vi "Fetch Measurement-Sweep.vi"(8 "error in (no error)":errorcluster, 10 "Measure Call Context in":refnum<class "Measure Call Context.lvclass">, 11 "Sweep fetch measurement control":T1={"Source Ganged Session Out"={"Ganged Config"=enum."Series", "Session List"=[], "Session Mode"=[], "Channel"=[]}, "Load Ganged Session Out"={"Ganged Config"=enum."Series", "Session List"=[], "Session Mode"=[], "Channel"=[]}, "Source sweep values"=[], "Source sweep points"=0, "Load sweep values"=[], "Load sweep points"=0, "Measurement Results"={"Status"="", "Source sweep points"=0, "Load sweep points"=0, "Source sweep values"=[], "Load sweep values"=[], "Source voltages"=[], "Source currents"=[], "Load voltages"=[], "Load currents"=[], "Eload status"=""}, "Load ganged/single"=FALSE, "Source ganged/single"=FALSE, "Source channel name"="", "Load channel name"="", "Source session out"="", "Load session out"="", "Load Source ON/OFF"=enum."SOURCE AND LOAD OFF", "Measurement timeout"=10.0} {"Measurement timeout" format="%.3p"}) -> (0 "error out":errorcluster, 3 "Sweep fetch measurement":T1={"Source Ganged Session Out"={"Ganged Config"=enum."Series", "Session List"=[], "Session Mode"=[], "Channel"=[]}, "Load Ganged Session Out"={"Ganged Config"=enum."Series", "Session List"=[], "Session Mode"=[], "Channel"=[]}, "Source sweep values"=[], "Source sweep points"=0, "Load sweep values"=[], "Load sweep points"=0, "Measurement Results"={"Status"="", "Source sweep points"=0, "Load sweep points"=0, "Source sweep values"=[], "Load sweep values"=[], "Source voltages"=[], "Source currents"=[], "Load voltages"=[], "Load currents"=[], "Eload status"=""}, "Load ganged/single"=FALSE, "Source ganged/single"=FALSE, "Source channel name"="", "Load channel name"="", "Source session out"="", "Load session out"="", "Load Source ON/OFF"=enum."SOURCE AND LOAD OFF", "Measurement timeout"=10.0} {"Measurement timeout" format="%.3p"})   [LabVIEW 2021, in "Sweep_Channel Ganging.lvlib"]
doc: "This vi fetches the measurement for the different configuration of single and ganging also when only source or load is enabled"
uses:
  Controls/Sweep fetch measurement control.ctl
  shared subVIs/ctl/NIDCPower_channel_ganging - ctl - ganged session.ctl
  shared subVIs/ctl/NIDCPower_channel_ganging - ctl - ganged config.ctl
  shared subVIs/ctl/NIDCPower_channel_ganging - ctl - channel mode.ctl
  Measurement Results.ctl
  <vilib>/Plug-In SDKs/Measurements/Measure Call Context/Measure Call Context.lvclass
  <vilib>/Plug-In SDKs/Measurements/Measure Call Context/Accessor/Is Canceled.vi
  Sweep_Channel Ganging.lvlib
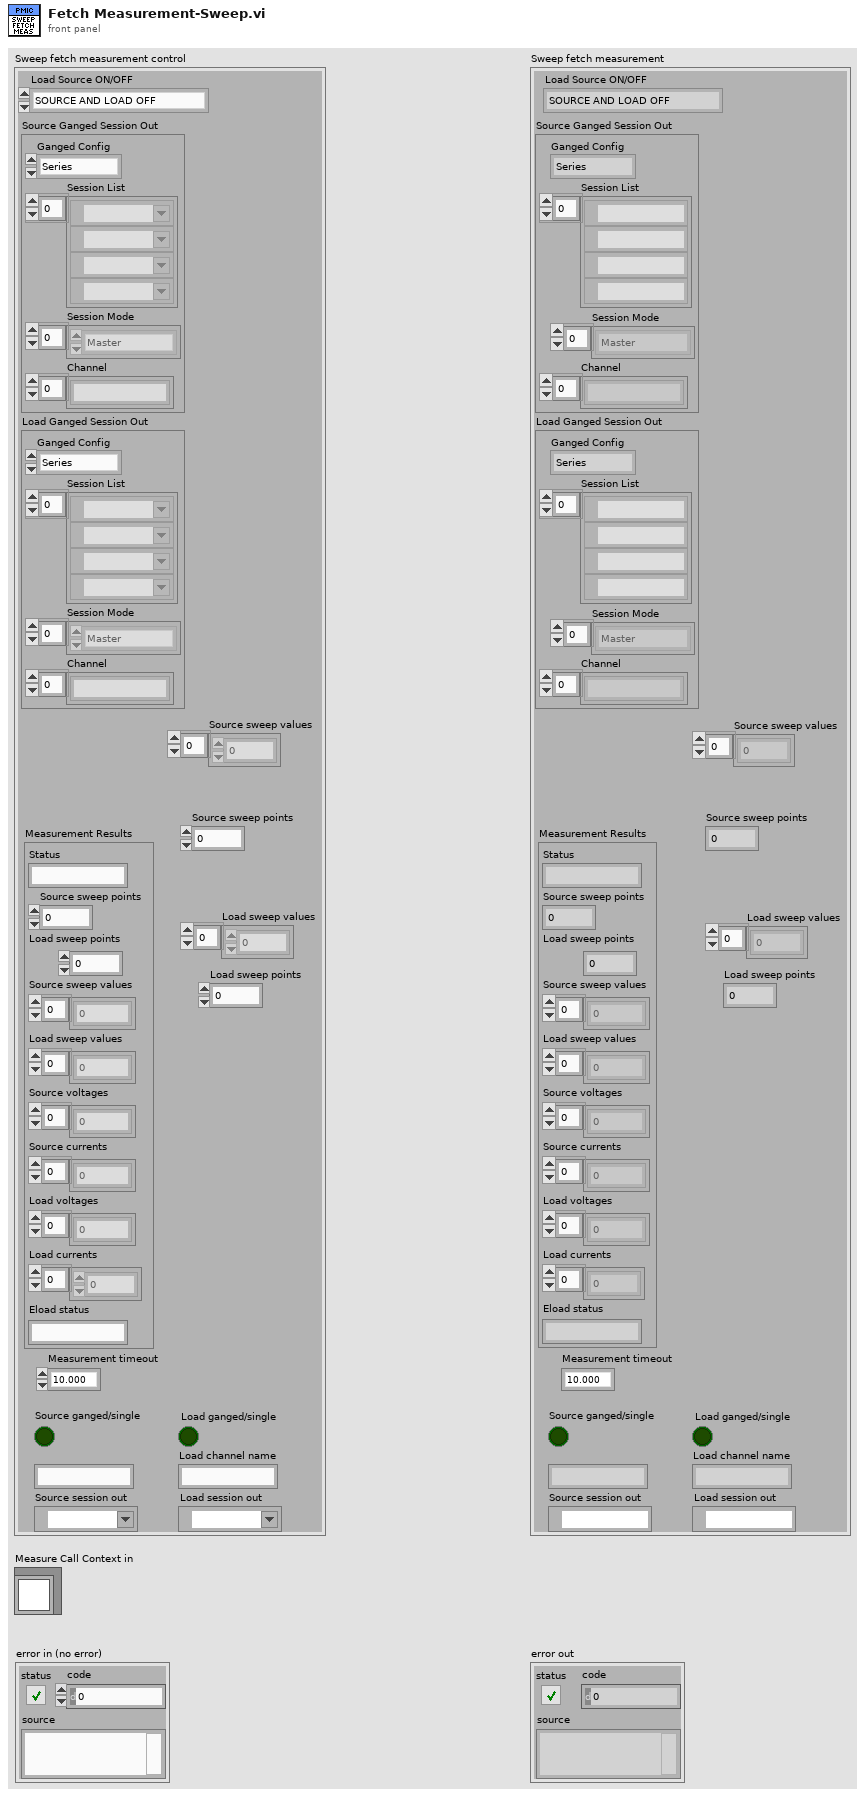
[diagram p1: front panel]
types:
  T1 = typedef "Sweep_Channel Ganging.lvlib/Sweep fetch measurement control.ctl" = cluster{"Source Ganged Session Out":T2, "Load Ganged Session Out":T2, "Source sweep values":dbl[], "Source sweep points":i32, "Load sweep values":dbl[], "Load sweep points":i32, "Measurement Results":T5, "Load ganged/single":bool, "Source ganged/single":bool, "Source channel name":string, "Load channel name":string, "Source session out":refnum<k15>, "Load session out":refnum<k15>, "Load Source ON/OFF":enum16{"SOURCE AND LOAD OFF", "SOURCE ON", "LOAD ON", "SOURCE AND LOAD ON"}, "Measurement timeout":dbl}
  T2 = typedef "NIDCPower_channel_ganging - ctl - ganged session.ctl" = cluster{"Ganged Config":T3, "Session List":refnum<k15>[], "Session Mode":T4[], "Channel":string[]}
  T3 = typedef "NIDCPower_channel_ganging - ctl - ganged config.ctl" = enum32{"Series", "Parallel", "Manual"}
  T4 = typedef "NIDCPower_channel_ganging - ctl - channel mode.ctl" = enum32{"Master", "Slave", "Slave - Inverted"}
  T5 = typedef "Sweep_Channel Ganging.lvlib/Measurement Results.ctl" = cluster{"Status":string, "Source sweep points":i32, "Load sweep points":i32, "Source sweep values":dbl[], "Load sweep values":dbl[], "Source voltages":dbl[], "Source currents":dbl[], "Load voltages":dbl[], "Load currents":dbl[], "Eload status":string}
  T6 = enum16{"SOURCE AND LOAD OFF", "SOURCE ON", "LOAD ON", "SOURCE AND LOAD ON"}
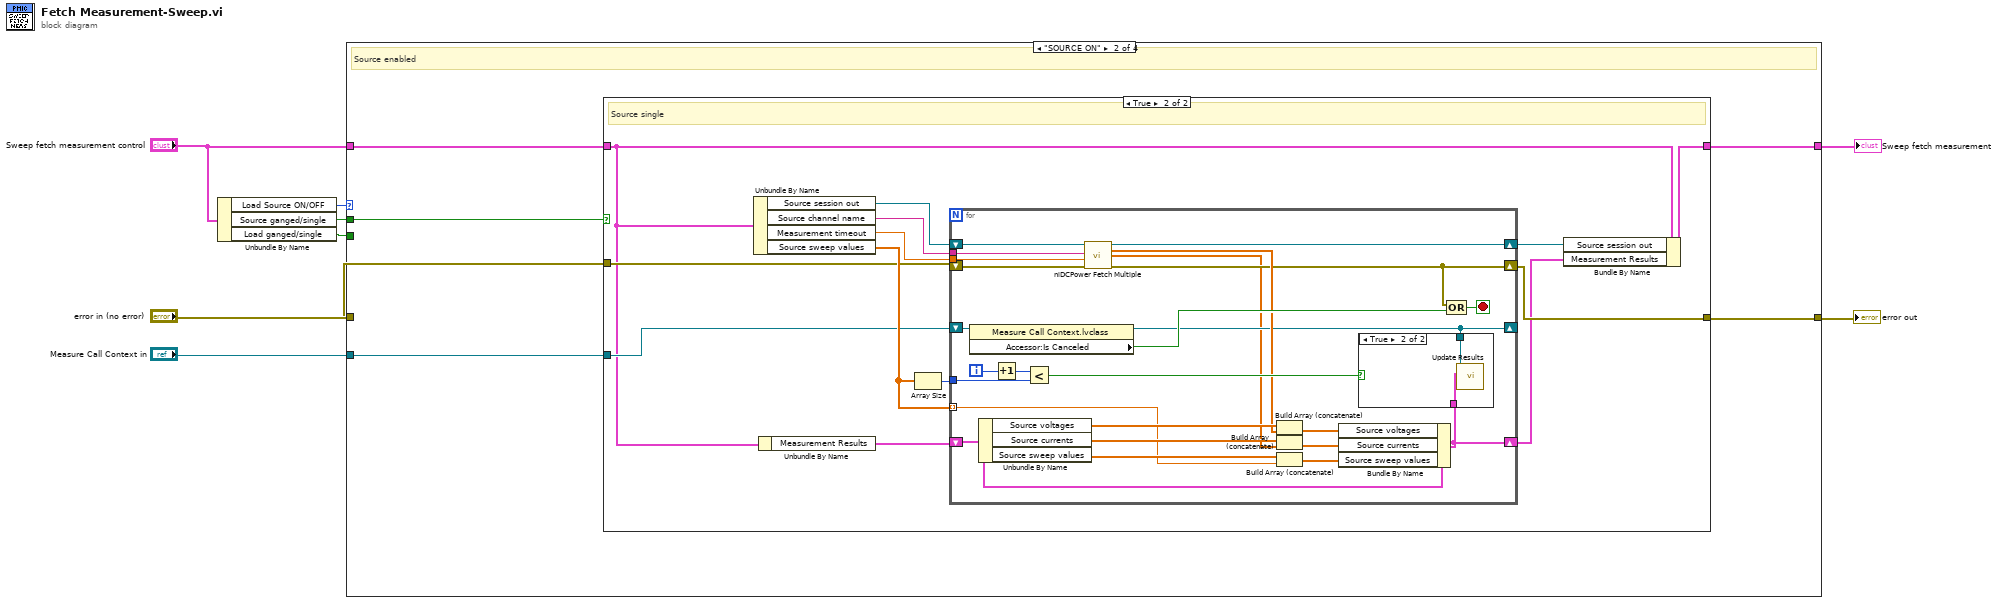
[diagram p0: block diagram]
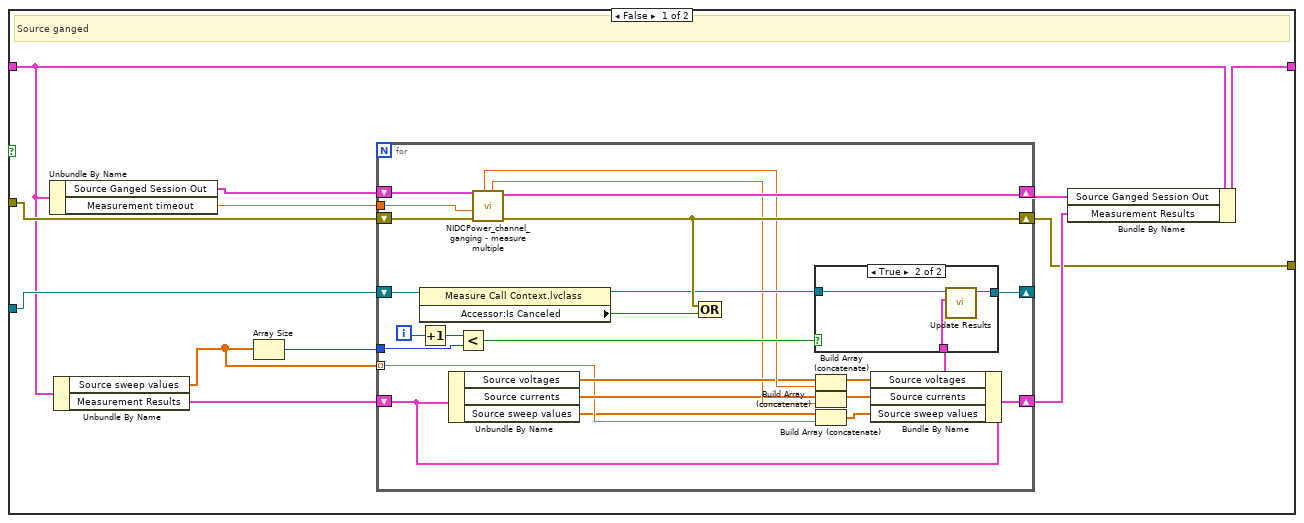
[diagram p3: hidden frame]
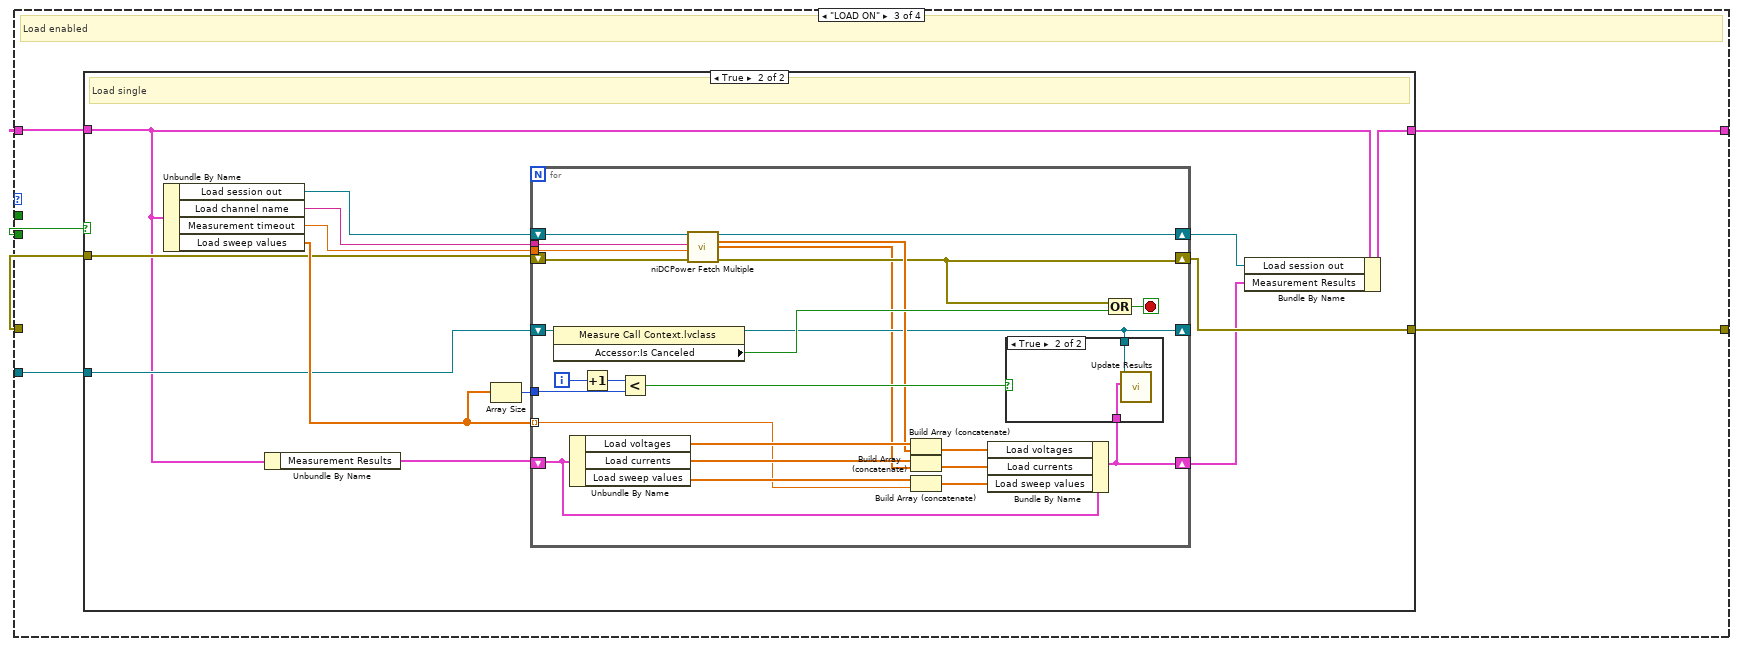
[diagram p6: hidden frame]
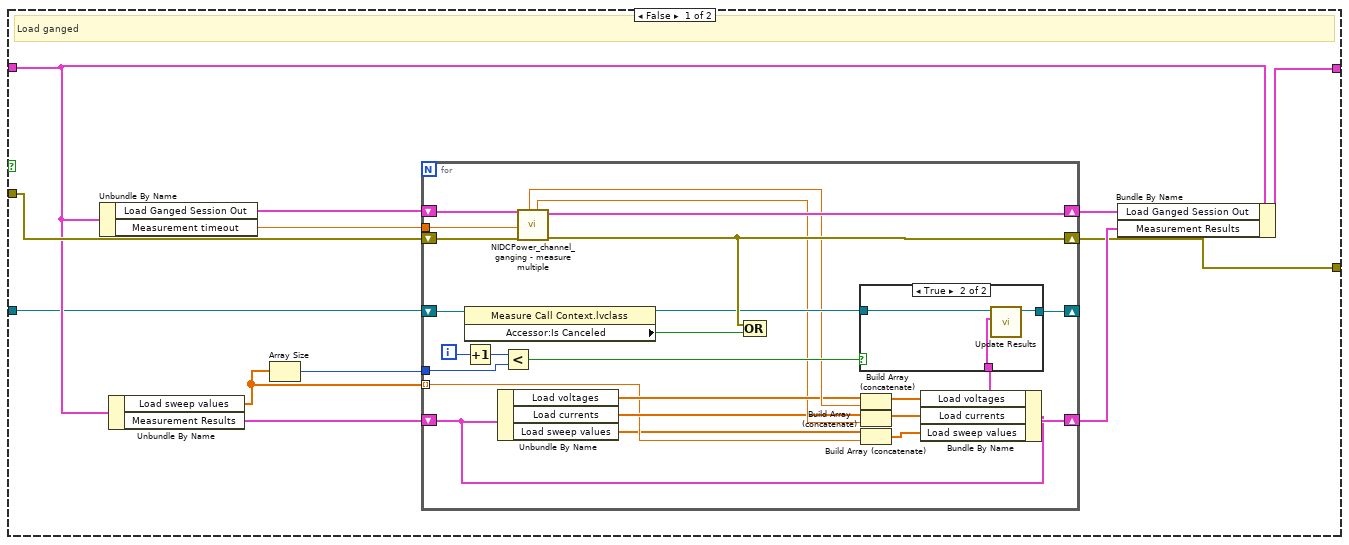
[diagram p7: hidden frame]
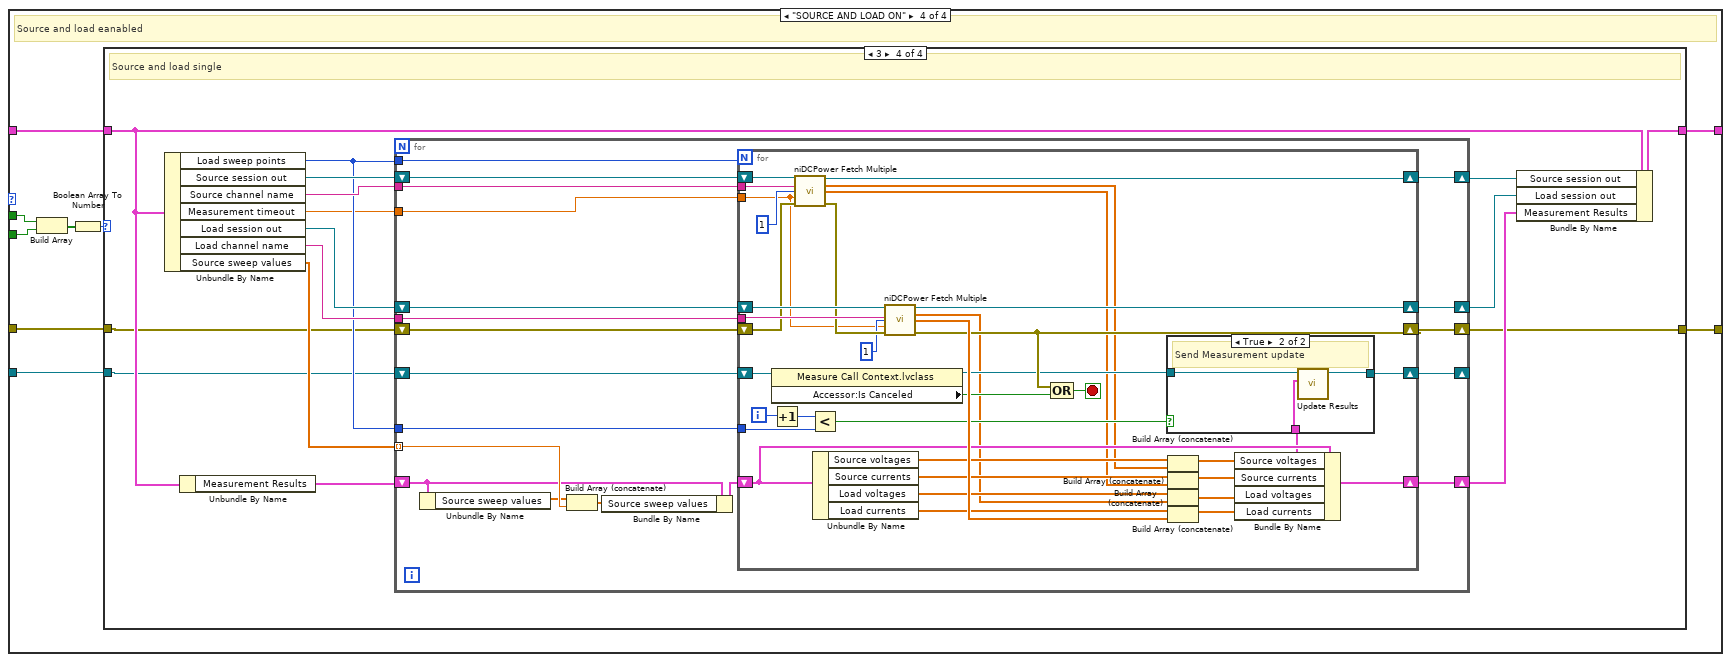
[diagram p10: hidden frame]
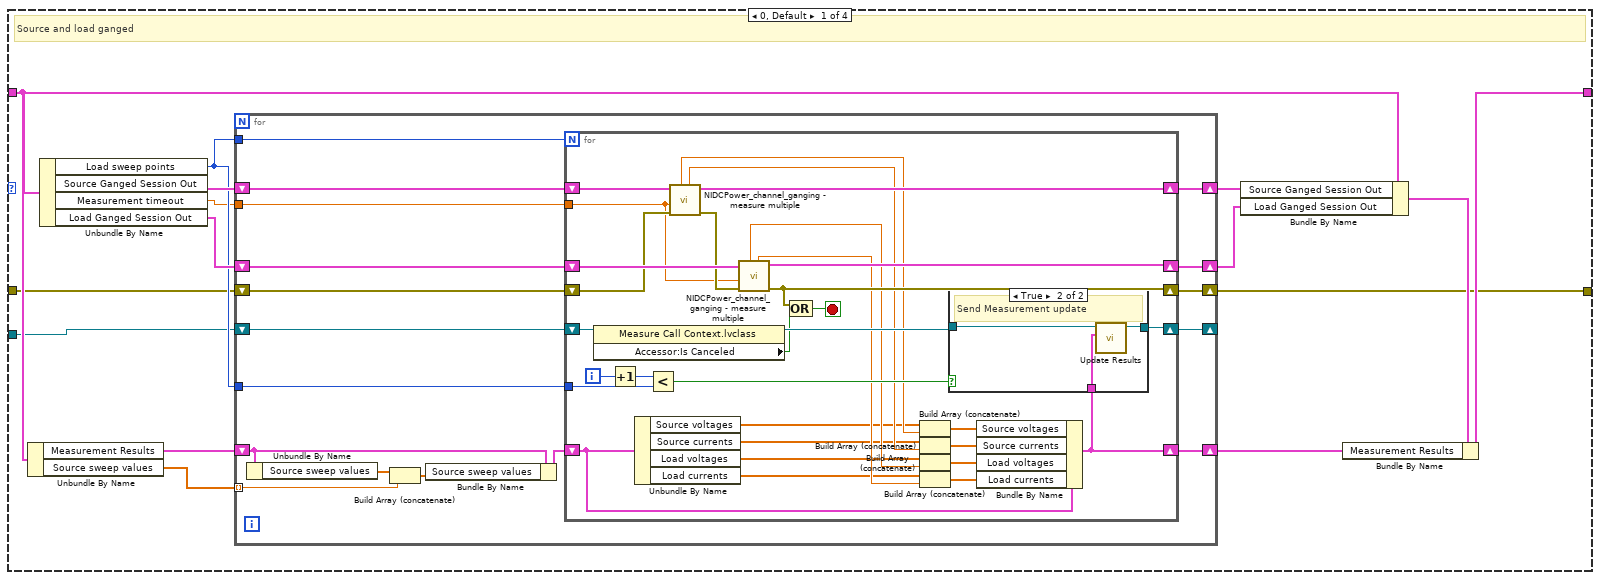
[diagram p11: hidden frame]
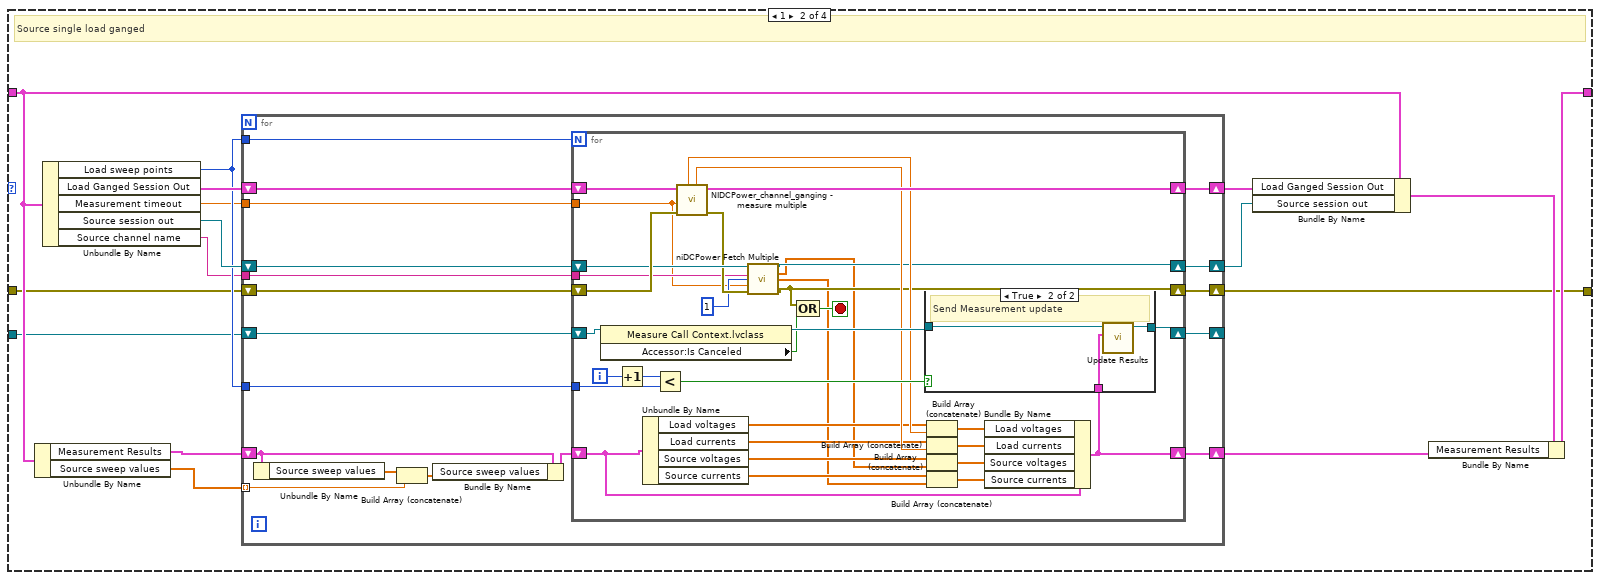
[diagram p13: hidden frame]
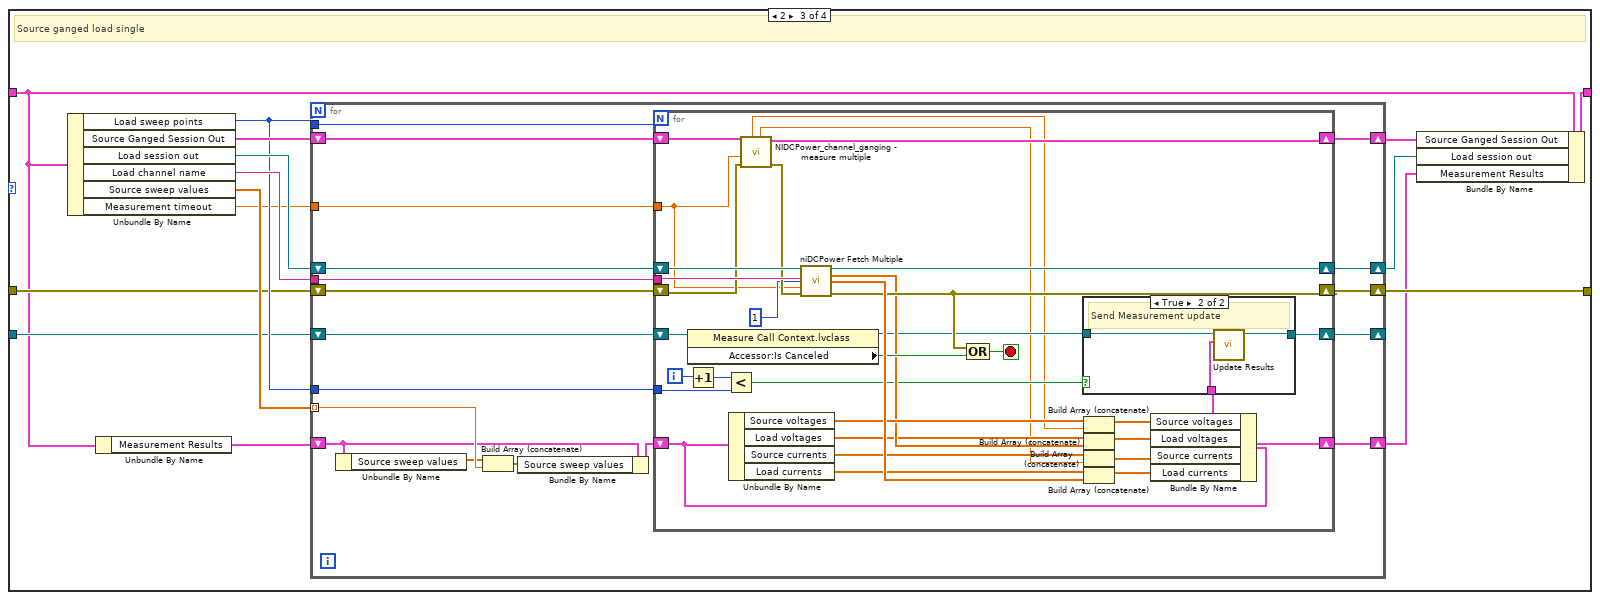
[diagram p15: hidden frame]
diagram:
  n1 = Unbundle By Name("Sweep fetch measurement control") -> ("Load Source ON/OFF"=w4:T6, "Source ganged/single"=w3:bool, "Load ganged/single"=w2:bool)
  n2 = case shown="\"SOURCE ON\"" w4 {
    tunnel: "Sweep fetch measurement control" -> [w10 w15 w100 w191]
    tunnel: [w10 w12 w98 w190] -> w1
    tunnel: "Measure Call Context in" -> [_ w13 w99 w189]
    tunnel: [w9 w11 w97 w188] -> w7
    tunnel: "error in (no error)" -> [w9 w16 w102 w187]
    tunnel: w3 -> [_ w14 _ w185]
    tunnel: w2 -> [_ _ w101 w184]
    frame "SOURCE AND LOAD OFF", Default {
      # "both disabled"
    }
    frame "SOURCE ON" {
      # "Source enabled"
      n3 = case shown="True" w14 {
        tunnel: w16 -> [w26 w65]
        tunnel: w15 -> [w23 w61]
        tunnel: w13 -> [w25 w63]
        tunnel: [w20 w60] -> w12
        tunnel: [w19 w62] -> w11
        frame False {
          # "Source ganged"
          n4 = Unbundle By Name(w23) -> ("Source Ganged Session Out"=w28:T2, "Measurement timeout"=w17:dbl)
          n5 = Unbundle By Name(w23) -> ("Source sweep values"=w18:dbl[], "Measurement Results"=w22:T5)
          n6 = Array Size(array=w18) -> (size(s)=w24:i32)
          n7 = for {
            shift-right: [w51] -> w19
            shift-left: w26 -> [w52]
            shift-right: [w50] -> w27
            shift-left: w28 -> [w49]
            shift-right: [w47] -> _
            shift-left: w25 -> [w48]
            shift-right: [w46] -> w21
            shift-left: w22 -> [w36]
            tunnel: w18 -> [w32] mode=indexing
            tunnel: w24 -> [w38]
            tunnel: w17 -> [w29]
            i -> [w37]
            n8 = property class="Measure Call Context.lvclass"(reference=w48) -> (reference out=w43:refnum<class "Measure Call Context.lvclass">, "Accessor:Is Canceled"=w45:bool)  [unwired: 1 in, 1 out]
            n9 = Increment(x=w37) -> (x+1=w44:i32)
            n10 = Unbundle By Name(w36) -> ("Source voltages"=w35:dbl[], "Source currents"=w33:dbl[], "Source sweep values"=w31:dbl[])
            n11 = Less?(x=w44, y=w38) -> (x < y?=w42:bool)
            n12 = call "NIDCPower_channel_ganging - measure multiple.vi"("error in (no error)"=w52, "timeout (1.0)"=w29, "Ganged Session In"=w49) -> ("error out"=w51:errorcluster, "Ganged Session Out"=w50:T2, "ganged current measurement"=w34:dbl, "ganged voltage measurement"=w39:dbl)  [unwired: 1 in, 4 out]
            n13 = Compound Arithmetic op=OR(w51, w45) -> ()  [unwired: 1 out]
            n14 = Build Array (concatenate)(w35, w39) -> (w41:dbl[])
            n15 = Build Array (concatenate)(w33, w34) -> (w40:dbl[])
            n16 = Build Array (concatenate)(w31, w32) -> (w30:dbl[])
            n17 = Bundle By Name(cluster=w36, "Source voltages"=w41, "Source currents"=w40, "Source sweep values"=w30) -> (w46:T5)
            n18 = case shown="True" w42 {
              tunnel: w43 -> [w53 w56]
              tunnel: [w53 w55] -> w47
              tunnel: w46 -> [_ w54]
              frame False {
              }
              frame True {
                n19 = call <vilib>:"Update Results.vi"("measurement results"=w54, "measure call context in"=w56) -> ("measure call context out"=w55:refnum<class "Measure Call Context.lvclass">)  [unwired: 8 in, 1 out]
              }
            }
          }
          n20 = Bundle By Name(cluster=w23, "Source Ganged Session Out"=w27, "Measurement Results"=w21) -> (w20:T1)
        }
        frame True {
          # "Source single"
          n21 = Unbundle By Name(w61) -> ("Source session out"=w69:refnum<k15>, "Source channel name"=w68:string, "Measurement timeout"=w57:dbl, "Source sweep values"=w67:dbl[])
          n22 = Unbundle By Name(w61) -> ("Measurement Results"=w64:T5)
          n23 = Array Size(array=w67) -> (size(s)=w66:i32)
          n24 = for {
            shift-right: [w75] -> w62
            shift-left: w65 -> [w92]
            shift-right: [w93] -> w59
            shift-left: w69 -> [w94]
            shift-right: [w84] -> w58
            shift-left: w64 -> [w85]
            shift-right: [w80] -> _
            shift-left: w63 -> [w81]
            tunnel: w68 -> [w79]
            tunnel: w67 -> [w71] mode=indexing
            tunnel: w66 -> [w78]
            tunnel: w57 -> [w70]
            i -> [w91]
            stop <- w87 stop-if-true
            n25 = property class="Measure Call Context.lvclass"(reference=w81) -> (reference out=w80:refnum<class "Measure Call Context.lvclass">, "Accessor:Is Canceled"=w88:bool)  [unwired: 1 in, 1 out]
            n26 = Unbundle By Name(w85) -> ("Source voltages"=w86:dbl[], "Source currents"=w77:dbl[], "Source sweep values"=w76:dbl[])
            n27 = Increment(x=w91) -> (x+1=w90:i32)
            n28 = Less?(x=w90, y=w78) -> (x < y?=w89:bool)
            n29 = call <instrlib>:"niDCPower Fetch Multiple.vi"("instrument handle"=w94, "channel name"=w79, "timeout (1.0)"=w70, "error in (no error)"=w92) -> ("instrument handle out"=w93:refnum<k15>, "voltage measurements"=w83:dbl[], "current measurements"=w72:dbl[], "error out"=w75:errorcluster)  [unwired: 1 in, 7 out]
            n30 = Build Array (concatenate)(w86, w83) -> (w73:dbl[])
            n31 = Build Array (concatenate)(w77, w72) -> (w74:dbl[])
            n32 = Build Array (concatenate)(w76, w71) -> (w82:dbl[])
            n33 = Bundle By Name(cluster=w85, "Source voltages"=w73, "Source currents"=w74, "Source sweep values"=w82) -> (w84:T5)
            n34 = case shown="True" w89 {
              tunnel: w80 -> [_ w96]
              tunnel: w84 -> [_ w95]
              frame False {
              }
              frame True {
                n35 = call <vilib>:"Update Results.vi"("measurement results"=w95, "measure call context in"=w96) -> ()  [unwired: 8 in, 2 out]
              }
            }
            n36 = Compound Arithmetic op=OR(w75, w88) -> (w87:bool)
          }
          n37 = Bundle By Name(cluster=w61, "Source session out"=w59, "Measurement Results"=w58) -> (w60:T1)
        }
      }
    }
    frame "LOAD ON" {
      # "Load enabled"
      n38 = case shown="True" w101 {
        tunnel: w102 -> [w112 w151]
        tunnel: w100 -> [w110 w147]
        tunnel: w99 -> [w105 w149]
        tunnel: [w107 w146] -> w98
        tunnel: [w106 w148] -> w97
        frame False {
          # "Load ganged"
          n39 = Unbundle By Name(w110) -> ("Load Ganged Session Out"=w114:T2, "Measurement timeout"=w104:dbl)
          n40 = Unbundle By Name(w110) -> ("Load sweep values"=w103:dbl[], "Measurement Results"=w109:T5)
          n41 = Array Size(array=w103) -> (size(s)=w111:i32)
          n42 = for {
            shift-right: [w137] -> w106
            shift-left: w112 -> [w138]
            shift-right: [w136] -> w113
            shift-left: w114 -> [w135]
            shift-right: [w133] -> _
            shift-left: w105 -> [w134]
            shift-right: [w132] -> w108
            shift-left: w109 -> [w122]
            tunnel: w103 -> [w118] mode=indexing
            tunnel: w111 -> [w124]
            tunnel: w104 -> [w115]
            i -> [w123]
            n43 = property class="Measure Call Context.lvclass"(reference=w134) -> (reference out=w129:refnum<class "Measure Call Context.lvclass">, "Accessor:Is Canceled"=w131:bool)  [unwired: 1 in, 1 out]
            n44 = Increment(x=w123) -> (x+1=w130:i32)
            n45 = Unbundle By Name(w122) -> ("Load voltages"=w121:dbl[], "Load currents"=w119:dbl[], "Load sweep values"=w117:dbl[])
            n46 = Less?(x=w130, y=w124) -> (x < y?=w128:bool)
            n47 = call "NIDCPower_channel_ganging - measure multiple.vi"("error in (no error)"=w138, "timeout (1.0)"=w115, "Ganged Session In"=w135) -> ("error out"=w137:errorcluster, "Ganged Session Out"=w136:T2, "ganged current measurement"=w120:dbl, "ganged voltage measurement"=w125:dbl)  [unwired: 1 in, 4 out]
            n48 = Compound Arithmetic op=OR(w137, w131) -> ()  [unwired: 1 out]
            n49 = Build Array (concatenate)(w121, w125) -> (w127:dbl[])
            n50 = Build Array (concatenate)(w119, w120) -> (w126:dbl[])
            n51 = Build Array (concatenate)(w117, w118) -> (w116:dbl[])
            n52 = Bundle By Name(cluster=w122, "Load voltages"=w127, "Load currents"=w126, "Load sweep values"=w116) -> (w132:T5)
            n53 = case shown="True" w128 {
              tunnel: w129 -> [w139 w142]
              tunnel: [w139 w141] -> w133
              tunnel: w132 -> [_ w140]
              frame False {
              }
              frame True {
                n54 = call <vilib>:"Update Results.vi"("measurement results"=w140, "measure call context in"=w142) -> ("measure call context out"=w141:refnum<class "Measure Call Context.lvclass">)  [unwired: 8 in, 1 out]
              }
            }
          }
          n55 = Bundle By Name(cluster=w110, "Load Ganged Session Out"=w113, "Measurement Results"=w108) -> (w107:T1)
        }
        frame True {
          # "Load single"
          n56 = Unbundle By Name(w147) -> ("Load session out"=w155:refnum<k15>, "Load channel name"=w154:string, "Measurement timeout"=w143:dbl, "Load sweep values"=w153:dbl[])
          n57 = Unbundle By Name(w147) -> ("Measurement Results"=w150:T5)
          n58 = Array Size(array=w153) -> (size(s)=w152:i32)
          n59 = for {
            shift-right: [w161] -> w148
            shift-left: w151 -> [w178]
            shift-right: [w179] -> w145
            shift-left: w155 -> [w180]
            shift-right: [w170] -> w144
            shift-left: w150 -> [w171]
            shift-right: [w166] -> _
            shift-left: w149 -> [w167]
            tunnel: w154 -> [w165]
            tunnel: w153 -> [w157] mode=indexing
            tunnel: w152 -> [w164]
            tunnel: w143 -> [w156]
            i -> [w177]
            stop <- w173 stop-if-true
            n60 = property class="Measure Call Context.lvclass"(reference=w167) -> (reference out=w166:refnum<class "Measure Call Context.lvclass">, "Accessor:Is Canceled"=w174:bool)  [unwired: 1 in, 1 out]
            n61 = Unbundle By Name(w171) -> ("Load voltages"=w172:dbl[], "Load currents"=w163:dbl[], "Load sweep values"=w162:dbl[])
            n62 = Increment(x=w177) -> (x+1=w176:i32)
            n63 = Less?(x=w176, y=w164) -> (x < y?=w175:bool)
            n64 = call <instrlib>:"niDCPower Fetch Multiple.vi"("instrument handle"=w180, "channel name"=w165, "timeout (1.0)"=w156, "error in (no error)"=w178) -> ("instrument handle out"=w179:refnum<k15>, "voltage measurements"=w169:dbl[], "current measurements"=w158:dbl[], "error out"=w161:errorcluster)  [unwired: 1 in, 7 out]
            n65 = Build Array (concatenate)(w172, w169) -> (w159:dbl[])
            n66 = Build Array (concatenate)(w163, w158) -> (w160:dbl[])
            n67 = Build Array (concatenate)(w162, w157) -> (w168:dbl[])
            n68 = Bundle By Name(cluster=w171, "Load voltages"=w159, "Load currents"=w160, "Load sweep values"=w168) -> (w170:T5)
            n69 = case shown="True" w175 {
              tunnel: w166 -> [_ w182]
              tunnel: w170 -> [_ w181]
              frame False {
              }
              frame True {
                n70 = call <vilib>:"Update Results.vi"("measurement results"=w181, "measure call context in"=w182) -> ()  [unwired: 8 in, 2 out]
              }
            }
            n71 = Compound Arithmetic op=OR(w161, w174) -> (w173:bool)
          }
          n72 = Bundle By Name(cluster=w147, "Load session out"=w145, "Measurement Results"=w144) -> (w146:T1)
        }
      }
    }
    frame "SOURCE AND LOAD ON" {
      # "Source and load eanabled"
      n73 = Build Array(w185, w184) -> (w186:bool[])
      n74 = Boolean Array To Number(Boolean array=w186) -> (number=w183:u32)
      n75 = case shown="3" w183 {
        tunnel: w191 -> [w202 w265 w335 w405]
        tunnel: [w198 w266 w334 w401] -> w190
        tunnel: w189 -> [w195 w264 w338 w403]
        tunnel: [w194 w262 w336 w402] -> w188
        tunnel: w187 -> [w193 w263 w339 w404]
        frame 0, Default {
          # "Source and load ganged"
          n76 = Unbundle By Name(w202) -> ("Measurement Results"=w196:T5, "Source sweep values"=w206:dbl[])
          n77 = Unbundle By Name(w202) -> ("Load sweep points"=w199:i32, "Source Ganged Session Out"=w200:T2, "Measurement timeout"=w192:dbl, "Load Ganged Session Out"=w201:T2)
          n78 = for {
            shift-right: [w222] -> w194
            shift-left: w193 -> [w223]
            shift-right: [w220] -> w204
            shift-left: w201 -> [w221]
            shift-right: [w218] -> w203
            shift-left: w200 -> [w219]
            shift-right: [w216] -> _
            shift-left: w195 -> [w217]
            shift-right: [w215] -> w197
            shift-left: w196 -> [w210]
            tunnel: w199 -> [w214]
            tunnel: w199 -> [w213]
            tunnel: w206 -> [w208] mode=indexing
            tunnel: w192 -> [w207]
            n79 = Unbundle By Name(w210) -> ("Source sweep values"=w212:dbl[])
            n80 = Build Array (concatenate)(w212, w208) -> (w211:dbl[])
            n81 = Bundle By Name(cluster=w210, "Source sweep values"=w211) -> (w209:T5)
            n82 = for {
              N: w213 -> [_]
              shift-right: [w243] -> w222
              shift-left: w223 -> [w252]
              shift-right: [w253] -> w220
              shift-left: w221 -> [w254]
              shift-right: [w249] -> w218
              shift-left: w219 -> [w250]
              shift-right: [w246] -> w216
              shift-left: w217 -> [w248]
              shift-right: [w239] -> w215
              shift-left: w209 -> [w242]
              tunnel: w214 -> [w229]
              tunnel: w207 -> [w224]
              i -> [w237]
              stop <- w245 stop-if-true
              n83 = property class="Measure Call Context.lvclass"(reference=w248) -> (reference out=w247:refnum<class "Measure Call Context.lvclass">, "Accessor:Is Canceled"=w244:bool)  [unwired: 1 in, 1 out]
              n84 = Increment(x=w237) -> (x+1=w238:i32)
              n85 = Unbundle By Name(w242) -> ("Source voltages"=w228:dbl[], "Source currents"=w227:dbl[], "Load voltages"=w226:dbl[], "Load currents"=w225:dbl[])
              n86 = Less?(x=w238, y=w229) -> (x < y?=w236:bool)
              n87 = call "NIDCPower_channel_ganging - measure multiple.vi"("error in (no error)"=w252, "timeout (1.0)"=w224, "Ganged Session In"=w250) -> ("error out"=w251:errorcluster, "Ganged Session Out"=w249:T2, "ganged current measurement"=w234:dbl, "ganged voltage measurement"=w235:dbl)  [unwired: 1 in, 4 out]
              n88 = call "NIDCPower_channel_ganging - measure multiple.vi"("error in (no error)"=w251, "timeout (1.0)"=w224, "Ganged Session In"=w254) -> ("error out"=w243:errorcluster, "Ganged Session Out"=w253:T2, "ganged current measurement"=w232:dbl, "ganged voltage measurement"=w233:dbl)  [unwired: 1 in, 4 out]
              n89 = Compound Arithmetic op=OR(w243, w244) -> (w245:bool)
              n90 = Build Array (concatenate)(w228, w235) -> (w241:dbl[])
              n91 = Build Array (concatenate)(w227, w234) -> (w240:dbl[])
              n92 = Build Array (concatenate)(w226, w233) -> (w231:dbl[])
              n93 = Build Array (concatenate)(w225, w232) -> (w230:dbl[])
              n94 = Bundle By Name(cluster=w242, "Source voltages"=w241, "Source currents"=w240, "Load voltages"=w231, "Load currents"=w230) -> (w239:T5)
              n95 = case shown="True" w236 {
                tunnel: w239 -> [_ w258]
                tunnel: w247 -> [w255 w257]
                tunnel: [w255 w256] -> w246
                frame False {
                  # "Doesn't send mesurement update"
                }
                frame True {
                  # "Send Measurement update"
                  n96 = call <vilib>:"Update Results.vi"("measurement results"=w258, "measure call context in"=w257) -> ("measure call context out"=w256:refnum<class "Measure Call Context.lvclass">)  [unwired: 8 in, 1 out]
                }
              }
            }
          }
          n97 = Bundle By Name(cluster=w202, "Source Ganged Session Out"=w203, "Load Ganged Session Out"=w204) -> (w205:T1)
          n98 = Bundle By Name(cluster=w205, "Measurement Results"=w197) -> (w198:T1)
        }
        frame 1 {
          # "Source single load ganged"
          n99 = Unbundle By Name(w265) -> ("Measurement Results"=w267:T5, "Source sweep values"=w274:dbl[])
          n100 = Unbundle By Name(w265) -> ("Load sweep points"=w269:i32, "Load Ganged Session Out"=w270:T2, "Measurement timeout"=w259:dbl, "Source session out"=w271:refnum<k15>, "Source channel name"=w260:string)
          n101 = for {
            shift-right: [w291] -> w262
            shift-left: w263 -> [w292]
            shift-right: [w289] -> w261
            shift-left: w271 -> [w290]
            shift-right: [w287] -> w272
            shift-left: w270 -> [w288]
            shift-right: [w285] -> _
            shift-left: w264 -> [w286]
            shift-right: [w284] -> w268
            shift-left: w267 -> [w279]
            tunnel: w269 -> [w283]
            tunnel: w269 -> [w282]
            tunnel: w274 -> [w277] mode=indexing
            tunnel: w260 -> [w276]
            tunnel: w259 -> [w275]
            n102 = Unbundle By Name(w279) -> ("Source sweep values"=w281:dbl[])
            n103 = Build Array (concatenate)(w281, w277) -> (w280:dbl[])
            n104 = Bundle By Name(cluster=w279, "Source sweep values"=w280) -> (w278:T5)
            n105 = for {
              N: w282 -> [_]
              shift-right: [w298] -> w291
              shift-left: w292 -> [w325]
              shift-right: [w300] -> w289
              shift-left: w290 -> [w301]
              shift-right: [w323] -> w287
              shift-left: w288 -> [w324]
              shift-right: [w320] -> w285
              shift-left: w286 -> [w322]
              shift-right: [w314] -> w284
              shift-left: w278 -> [w317]
              tunnel: w283 -> [w306]
              tunnel: w276 -> [w294]
              tunnel: w275 -> [w293]
              i -> [w312]
              stop <- w319 stop-if-true
              n106 = property class="Measure Call Context.lvclass"(reference=w322) -> (reference out=w321:refnum<class "Measure Call Context.lvclass">, "Accessor:Is Canceled"=w318:bool)  [unwired: 1 in, 1 out]
              n107 = Increment(x=w312) -> (x+1=w313:i32)
              n108 = Unbundle By Name(w317) -> ("Load voltages"=w305:dbl[], "Load currents"=w304:dbl[], "Source voltages"=w303:dbl[], "Source currents"=w302:dbl[])
              n109 = Less?(x=w313, y=w306) -> (x < y?=w311:bool)
              n110 = call "NIDCPower_channel_ganging - measure multiple.vi"("error in (no error)"=w325, "timeout (1.0)"=w293, "Ganged Session In"=w324) -> ("error out"=w299:errorcluster, "Ganged Session Out"=w323:T2, "ganged current measurement"=w309:dbl, "ganged voltage measurement"=w310:dbl)  [unwired: 1 in, 4 out]
              n111 = call <instrlib>:"niDCPower Fetch Multiple.vi"("instrument handle"=w301, "channel name"=w294, "count (1)"=1, "timeout (1.0)"=w293, "error in (no error)"=w299) -> ("instrument handle out"=w300:refnum<k15>, "voltage measurements"=w297:dbl[], "current measurements"=w296:dbl[], "error out"=w298:errorcluster)  [unwired: 7 out]
              n112 = Compound Arithmetic op=OR(w298, w318) -> (w319:bool)
              n113 = Build Array (concatenate)(w305, w310) -> (w316:dbl[])
              n114 = Build Array (concatenate)(w304, w309) -> (w315:dbl[])
              n115 = Build Array (concatenate)(w303, w297) -> (w308:dbl[])
              n116 = Build Array (concatenate)(w302, w296) -> (w307:dbl[])
              n117 = Bundle By Name(cluster=w317, "Load voltages"=w316, "Load currents"=w315, "Source voltages"=w308, "Source currents"=w307) -> (w314:T5)
              n118 = case shown="True" w311 {
                tunnel: w314 -> [_ w329]
                tunnel: w321 -> [w326 w328]
                tunnel: [w326 w327] -> w320
                frame False {
                  # "Doesn't send mesurement update"
                }
                frame True {
                  # "Send Measurement update"
                  n119 = call <vilib>:"Update Results.vi"("measurement results"=w329, "measure call context in"=w328) -> ("measure call context out"=w327:refnum<class "Measure Call Context.lvclass">)  [unwired: 8 in, 1 out]
                }
              }
            }
          }
          n120 = Bundle By Name(cluster=w265, "Load Ganged Session Out"=w272, "Source session out"=w261) -> (w273:T1)
          n121 = Bundle By Name(cluster=w273, "Measurement Results"=w268) -> (w266:T1)
        }
        frame 2 {
          # "Source ganged load single"
          n122 = Unbundle By Name(w335) -> ("Load sweep points"=w340:i32, "Source Ganged Session Out"=w344:T2, "Load session out"=w343:refnum<k15>, "Load channel name"=w342:string, "Source sweep values"=w341:dbl[], "Measurement timeout"=w330:dbl)
          n123 = Unbundle By Name(w335) -> ("Measurement Results"=w337:T5)
          n124 = for {
            tunnel: w342 -> [w356]
            tunnel: w340 -> [w355]
            shift-right: [w361] -> w336
            shift-left: w339 -> [w362]
            shift-right: [w359] -> w332
            shift-left: w344 -> [w358]
            shift-right: [w360] -> w333
            shift-left: w343 -> [w357]
            shift-right: [w353] -> _
            shift-left: w338 -> [w354]
            shift-right: [w346] -> w331
            shift-left: w337 -> [w350]
            tunnel: w341 -> [w351] mode=indexing
            tunnel: w340 -> [w352]
            tunnel: w330 -> [w345]
            n125 = Unbundle By Name(w350) -> ("Source sweep values"=w347:dbl[])
            n126 = Build Array (concatenate)(w347, w351) -> (w348:dbl[])
            n127 = Bundle By Name(cluster=w350, "Source sweep values"=w348) -> (w349:T5)
            n128 = for {
              N: w355 -> [_]
              tunnel: w356 -> [w394]
              shift-right: [w395] -> w360
              shift-left: w357 -> [w393]
              shift-right: [w390] -> w361
              shift-left: w362 -> [w370]
              shift-right: [w367] -> w359
              shift-left: w358 -> [w368]
              shift-right: [w380] -> w353
              shift-left: w354 -> [w387]
              shift-right: [w371] -> w346
              shift-left: w349 -> [w372]
              tunnel: w352 -> [w379]
              tunnel: w345 -> [w363]
              i -> [w388]
              stop <- w382 stop-if-true
              n129 = property class="Measure Call Context.lvclass"(reference=w387) -> (reference out=w381:refnum<class "Measure Call Context.lvclass">, "Accessor:Is Canceled"=w391:bool)  [unwired: 1 in, 1 out]
              n130 = Increment(x=w388) -> (x+1=w389:i32)
              n131 = Less?(x=w389, y=w379) -> (x < y?=w376:bool)
              n132 = Unbundle By Name(w372) -> ("Source voltages"=w384:dbl[], "Load voltages"=w377:dbl[], "Source currents"=w378:dbl[], "Load currents"=w385:dbl[])
              n133 = call "NIDCPower_channel_ganging - measure multiple.vi"("error in (no error)"=w370, "timeout (1.0)"=w363, "Ganged Session In"=w368) -> ("error out"=w369:errorcluster, "Ganged Session Out"=w367:T2, "ganged current measurement"=w365:dbl, "ganged voltage measurement"=w366:dbl)  [unwired: 1 in, 4 out]
              n134 = call <instrlib>:"niDCPower Fetch Multiple.vi"("instrument handle"=w393, "channel name"=w394, "count (1)"=1, "timeout (1.0)"=w363, "error in (no error)"=w369) -> ("instrument handle out"=w395:refnum<k15>, "voltage measurements"=w383:dbl[], "current measurements"=w392:dbl[], "error out"=w390:errorcluster)  [unwired: 7 out]
              n135 = Compound Arithmetic op=OR(w390, w391) -> (w382:bool)
              n136 = Build Array (concatenate)(w384, w366) -> (w375:dbl[])
              n137 = Build Array (concatenate)(w377, w383) -> (w374:dbl[])
              n138 = Build Array (concatenate)(w378, w365) -> (w386:dbl[])
              n139 = Build Array (concatenate)(w385, w392) -> (w373:dbl[])
              n140 = Bundle By Name(cluster=w372, "Source voltages"=w375, "Load voltages"=w374, "Source currents"=w386, "Load currents"=w373) -> (w371:T5)
              n141 = case shown="True" w376 {
                tunnel: w381 -> [w396 w399]
                tunnel: [w396 w398] -> w380
                tunnel: w371 -> [_ w397]
                frame False {
                  # "Doesn't send mesurement update"
                }
                frame True {
                  # "Send Measurement update"
                  n142 = call <vilib>:"Update Results.vi"("measurement results"=w397, "measure call context in"=w399) -> ("measure call context out"=w398:refnum<class "Measure Call Context.lvclass">)  [unwired: 8 in, 1 out]
                }
              }
            }
          }
          n143 = Bundle By Name(cluster=w335, "Source Ganged Session Out"=w332, "Load session out"=w333, "Measurement Results"=w331) -> (w334:T1)
        }
        frame 3 {
          # "Source and load single"
          n144 = Unbundle By Name(w405) -> ("Load sweep points"=w410:i32, "Source session out"=w415:refnum<k15>, "Source channel name"=w414:string, "Measurement timeout"=w400:dbl, "Load session out"=w413:refnum<k15>, "Load channel name"=w412:string, "Source sweep values"=w411:dbl[])
          n145 = Unbundle By Name(w405) -> ("Measurement Results"=w409:T5)
          n146 = for {
            tunnel: w414 -> [w429]
            tunnel: w412 -> [w427]
            tunnel: w410 -> [w426]
            shift-right: [w433] -> w402
            shift-left: w404 -> [w434]
            shift-right: [w431] -> w407
            shift-left: w415 -> [w430]
            shift-right: [w432] -> w408
            shift-left: w413 -> [w428]
            shift-right: [w424] -> _
            shift-left: w403 -> [w425]
            shift-right: [w417] -> w406
            shift-left: w409 -> [w421]
            tunnel: w411 -> [w422] mode=indexing
            tunnel: w410 -> [w423]
            tunnel: w400 -> [w416]
            n147 = Unbundle By Name(w421) -> ("Source sweep values"=w418:dbl[])
            n148 = Build Array (concatenate)(w418, w422) -> (w419:dbl[])
            n149 = Bundle By Name(cluster=w421, "Source sweep values"=w419) -> (w420:T5)
            n150 = for {
              N: w426 -> [_]
              tunnel: w427 -> [w468]
              tunnel: w429 -> [w442]
              shift-right: [w469] -> w432
              shift-left: w428 -> [w467]
              shift-right: [w464] -> w433
              shift-left: w434 -> [w445]
              shift-right: [w440] -> w431
              shift-left: w430 -> [w443]
              shift-right: [w455] -> w424
              shift-left: w425 -> [w461]
              shift-right: [w446] -> w417
              shift-left: w420 -> [w447]
              tunnel: w423 -> [w454]
              tunnel: w416 -> [w435]
              i -> [w462]
              stop <- w457 stop-if-true
              n151 = property class="Measure Call Context.lvclass"(reference=w461) -> (reference out=w456:refnum<class "Measure Call Context.lvclass">, "Accessor:Is Canceled"=w465:bool)  [unwired: 1 in, 1 out]
              n152 = Increment(x=w462) -> (x+1=w463:i32)
              n153 = call <instrlib>:"niDCPower Fetch Multiple.vi"("instrument handle"=w443, "channel name"=w442, "count (1)"=1, "timeout (1.0)"=w435, "error in (no error)"=w445) -> ("instrument handle out"=w440:refnum<k15>, "voltage measurements"=w441:dbl[], "current measurements"=w437:dbl[], "error out"=w444:errorcluster)  [unwired: 7 out]
              n154 = Less?(x=w463, y=w454) -> (x < y?=w451:bool)
              n155 = Unbundle By Name(w447) -> ("Source voltages"=w458:dbl[], "Source currents"=w452:dbl[], "Load voltages"=w453:dbl[], "Load currents"=w459:dbl[])
              n156 = call <instrlib>:"niDCPower Fetch Multiple.vi"("instrument handle"=w467, "channel name"=w468, "count (1)"=1, "timeout (1.0)"=w435, "error in (no error)"=w444) -> ("instrument handle out"=w469:refnum<k15>, "voltage measurements"=w436:dbl[], "current measurements"=w466:dbl[], "error out"=w464:errorcluster)  [unwired: 7 out]
              n157 = Compound Arithmetic op=OR(w464, w465) -> (w457:bool)
              n158 = Build Array (concatenate)(w458, w441) -> (w450:dbl[])
              n159 = Build Array (concatenate)(w452, w437) -> (w449:dbl[])
              n160 = Build Array (concatenate)(w453, w436) -> (w460:dbl[])
              n161 = Build Array (concatenate)(w459, w466) -> (w448:dbl[])
              n162 = Bundle By Name(cluster=w447, "Source voltages"=w450, "Source currents"=w449, "Load voltages"=w460, "Load currents"=w448) -> (w446:T5)
              n163 = case shown="True" w451 {
                tunnel: w456 -> [w470 w473]
                tunnel: [w470 w472] -> w455
                tunnel: w446 -> [_ w471]
                frame False {
                  # "Doesn't send mesurement update"
                }
                frame True {
                  # "Send Measurement update"
                  n164 = call <vilib>:"Update Results.vi"("measurement results"=w471, "measure call context in"=w473) -> ("measure call context out"=w472:refnum<class "Measure Call Context.lvclass">)  [unwired: 8 in, 1 out]
                }
              }
            }
          }
          n165 = Bundle By Name(cluster=w405, "Source session out"=w407, "Load session out"=w408, "Measurement Results"=w406) -> (w401:T1)
        }
      }
    }
  }
  "error out" <- w7
  "Sweep fetch measurement" <- w1
